vi "Find Suit.vi"(6 "SS Path":path, 7 "error in (no error)":errorcluster, 10 "ROI 1st Card":T1) -> (0 "error out":errorcluster, 2 "Suit Score":dbl, 3 "Suit of Card":T2=enum."Unknown")   [LabVIEW 2015]
doc: "This VI checks the area in the ROI for a Club, Diamond, Heart, and Spade. In that order. As soon as one of these is found, the loop exits."
uses:
  Suit Enum.ctl
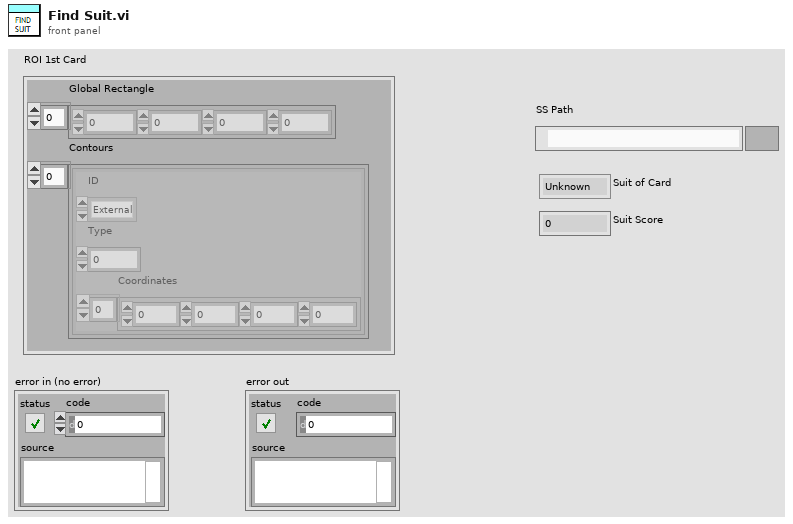
[diagram p1: front panel]
types:
  T1 = cluster{"Global Rectangle":i32[], "Contours":cluster{"ID":enum32{"External", "Internal"}, "Type":u32, "Coordinates":i32[]}[]}
  T2 = typedef "Suit Enum.ctl" = enum16{"Club", "Diamond", "Heart", "Spade", "Unknown"}
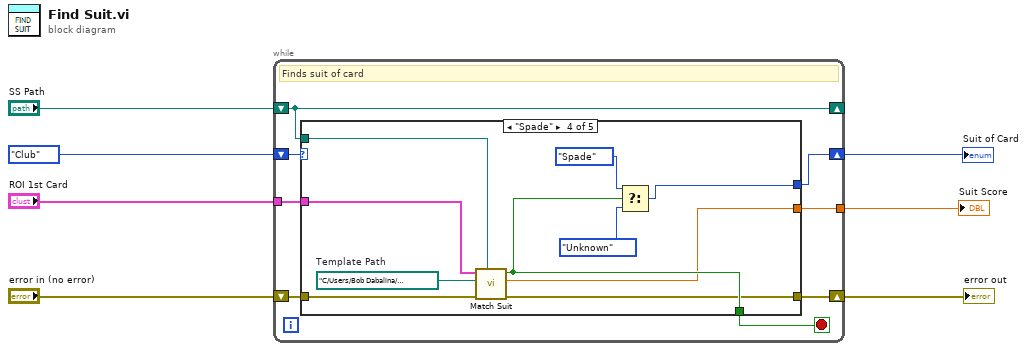
[diagram p0: block diagram]
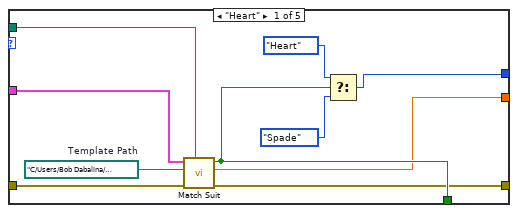
[diagram p2: hidden frame]
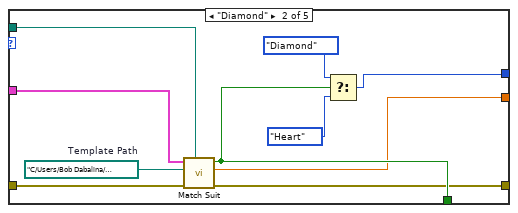
[diagram p3: hidden frame]
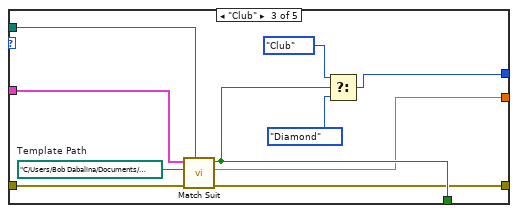
[diagram p4: hidden frame]
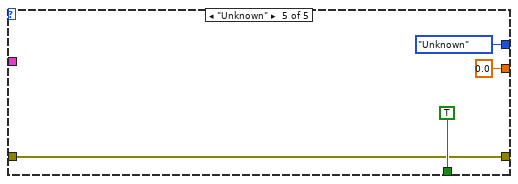
[diagram p5: hidden frame]
diagram:
  n1 = while {
    tunnel: "ROI 1st Card" -> [w15]
    shift-right: [w11] -> w5
    shift-left: "error in (no error)" -> [w14]
    shift-right: [w13] -> _
    shift-left: "SS Path" -> [w13]
    shift-right: [w9] -> w3
    shift-left: Suit_Enum."Club" ("Suit Card 1") -> [w10]
    tunnel: [w8] -> w1
    stop <- w12 stop-if-true
    # "Finds suit of card"
    n2 = case shown="\"Spade\"" w10 {
      tunnel: w15 -> [w25 w35 w45 w55 _]
      tunnel: w14 -> [w22 w32 w42 w52 w57]
      tunnel: w13 -> [w18 w28 w38 w48 _]
      tunnel: [w24 w34 w44 w54 Suit_Enum."Unknown" ("Suit Card 1")] -> w9
      tunnel: [w23 w33 w43 w53 TRUE ("Found Heart")] -> w12
      tunnel: [w21 w31 w41 w51 w57] -> w11
      tunnel: [w16 w26 w36 w46 0.0 ("Suit Score")] -> w8
      frame "Heart" {
        w17 = path "C:/Users/Bob Dabalina/Documents/Labview/Poker Hand2/Heart Template.png"  # Template Path
        n3 = call "Match Suit.vi"("SS Image Path"=w18, "error in"=w22, "Suit Template"=w17, "ROI Descriptor"=w25) -> ("error out"=w21:errorcluster, "Suit Score"=w16:dbl, "Suit Found?"=w23:bool)  [unwired: 5 in]
        n4 = Select(t=Suit_Enum."Heart" ("Suit Card 1"), s=w23, f=Suit_Enum."Spade" ("Suit Card 1")) -> (s? t:f=w24:T2)
      }
      frame "Diamond" {
        w27 = path "C:/Users/Bob Dabalina/Documents/Labview/Poker Hand2/Diamond Template.png"  # Template Path
        n5 = call "Match Suit.vi"("SS Image Path"=w28, "error in"=w32, "Suit Template"=w27, "ROI Descriptor"=w35) -> ("error out"=w31:errorcluster, "Suit Score"=w26:dbl, "Suit Found?"=w33:bool)  [unwired: 5 in]
        n6 = Select(t=Suit_Enum."Diamond" ("Suit Card 1"), s=w33, f=Suit_Enum."Heart" ("Suit Card 1")) -> (s? t:f=w34:T2)
      }
      frame "Club" {
        w37 = path "C:/Users/Bob Dabalina/Documents/Labview/Poker Hand2/Club Template.png"  # Template Path
        n7 = call "Match Suit.vi"("SS Image Path"=w38, "error in"=w42, "Suit Template"=w37, "ROI Descriptor"=w45) -> ("error out"=w41:errorcluster, "Suit Score"=w36:dbl, "Suit Found?"=w43:bool)  [unwired: 5 in]
        n8 = Select(t=Suit_Enum."Club" ("Suit Card 1"), s=w43, f=Suit_Enum."Diamond" ("Suit Card 1")) -> (s? t:f=w44:T2)
      }
      frame "Spade" {
        w47 = path "C:/Users/Bob Dabalina/Documents/Labview/Poker Hand2/Spade Template.png"  # Template Path
        n9 = call "Match Suit.vi"("SS Image Path"=w48, "error in"=w52, "Suit Template"=w47, "ROI Descriptor"=w55) -> ("error out"=w51:errorcluster, "Suit Score"=w46:dbl, "Suit Found?"=w53:bool)  [unwired: 5 in]
        n10 = Select(t=Suit_Enum."Spade" ("Suit Card 1"), s=w53, f=Suit_Enum."Unknown" ("Suit Card 1")) -> (s? t:f=w54:T2)
      }
      frame "Unknown" {
      }
    }
  }
  "Suit of Card" <- w3
  "error out" <- w5
  "Suit Score" <- w1
